vi "WFT AIO Enable Set.vi"(8 "Error In":errorcluster, 10 "fMasterEnable":bool, 11 "WaveForms Session In":T1) -> (0 "Error Out":errorcluster, 2 "ret":i32, 3 "WaveForms Session Out":T1)   [LabVIEW 2020, in "lv_waveforms_toolkit.lvlib"]
uses:
  lv_waveforms_toolkit.lvlib
  WFT Session.ctl
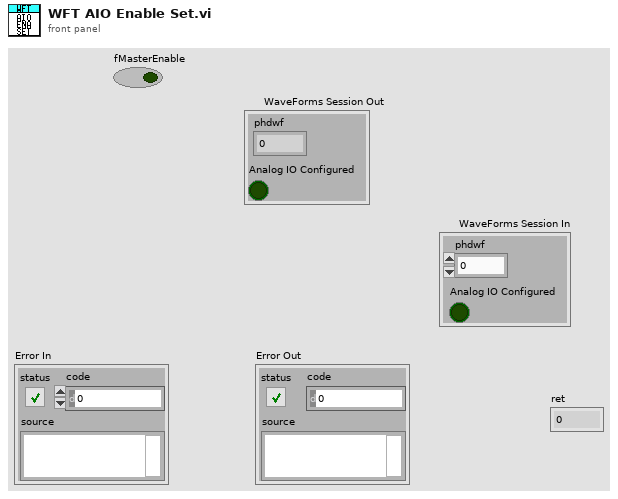
[diagram p1: front panel]
types:
  T1 = typedef "lv_waveforms_toolkit.lvlib/WFT Session.ctl" = cluster{"phdwf":i32, "Analog IO Configured":bool}
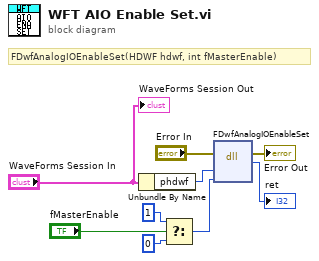
[diagram p0: block diagram]
diagram:
  # "FDwfAnalogIOEnableSet(HDWF hdwf, int fMasterEnable)"
  n1 = Unbundle By Name("WaveForms Session In") -> ("phdwf"=w5:i32)
  n2 = Select(t=1, s="fMasterEnable", f=0) -> (s? t:f=w1:i32)
  n3 = dll-call lib="dwf" fn="FDwfAnalogIOEnableSet"(error in="Error In", "phdwf"=w5, "fMasterEnable"=w1) -> (error out=→"Error Out":errorcluster, "return type"=→"ret":i32)  [unwired: 4 in, 1 out]
  "WaveForms Session Out" <- "WaveForms Session In"
